vi "getFileLastModifyTime.vi"(11 "path":path) -> (2 "date/time string":string)   [LabVIEW 2012]
panel:
  out "string":string
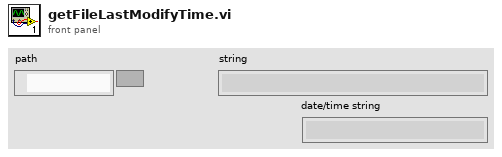
[diagram p1: front panel]
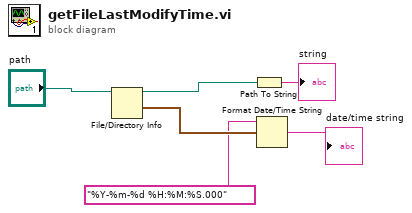
[diagram p0: block diagram]
diagram:
  n1 = File/Directory Info(path="path") -> (path out=w6:path, last mod=w5:timestamp)  [unwired: 1 in, 5 out]
  n2 = Path To String(path=w6) -> (string=→"string":string)
  n3 = Format Date/Time String(time format string (%c)="%Y-%m-%d %H:%M:%S.000", seconds (now)=w5) -> (date/time string=→"date/time string":string)  [unwired: 1 in]
